vi "Actor Core.vi"(8 "error in":errorcluster, 11 "Autosampler in":refnum<class "Autosampler.lvclass">) -> (0 "error out":errorcluster, 3 "Actor out":refnum<class "Actor.lvclass">)   [LabVIEW 2023, in "Autosampler.lvlib" / "Autosampler.lvclass"]
doc: "(<B>Filename</B>: Actor Framework.lvlib:Actor.lvclass:Actor Core.vi)\n\nReceives messages to the actor, reacts to them, and initiates any error handling that may shut the actor down.\n\nDescendant classes may override this VI to append parallel tasks for the actor to complete while it handles messages. Overrides use the Call Parent Method node."
uses:
  Autosampler.lvclass
  Autosampler.lvclass/Autosampler.ctl
  Device/Device.lvclass
  <vilib>/ActorFramework/Actor/Actor.lvclass
  C:/FLASH/Development/Hardware/Device/Device.lvclass
  C:/Program Files/National Instruments/LabVIEW 2023/vi.lib/ActorFramework/Actor/Actor.lvclass
  C:/FLASH/Development/Hardware/Autosampler/Autosampler.lvclass
  Autosampler Messages/Status Update Msg/Status Update Msg.lvclass
  <vilib>/ActorFramework/Message Enqueuer/Message Priority.ctl
  <vilib>/ActorFramework/Message Enqueuer/Message Enqueuer.lvclass
panel:
  in  "Stop Button":bool
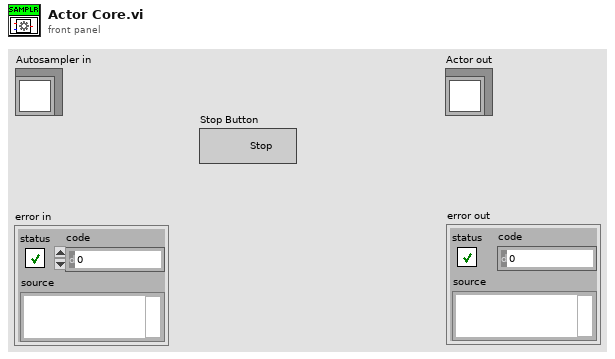
[diagram p1: front panel]
types:
  T1 = typedef "Actor Framework.lvlib/Message Enqueuer.lvclass/Message Priority.ctl" = enum16{"Low", "Normal", "High"}
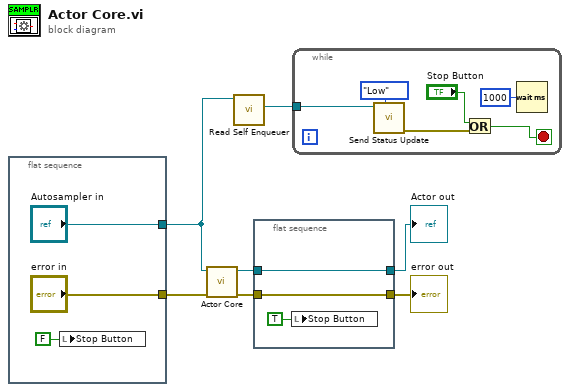
[diagram p0: block diagram]
diagram:
  n1 = flat-sequence {
    tunnel: ["error in"] -> w7
    tunnel: ["Autosampler in"] -> w2
    frame #0 {
      n2 = local write "Stop Button"(FALSE ("Stop Button")) -> ()
    }
  }
  n3 = call-parent "Actor Core.vi"("error in"=w7, "Device in"=w2) -> ("error out"=w3:errorcluster, "Actor out"=w6:refnum<class "Actor.lvclass">)  [unwired: 8 in]
  n4 = call <vilib>:"Read Self Enqueuer.vi"("Actor"=w2) -> ("Self Enqueuer"=w1:refnum<class "Message Enqueuer.lvclass">)  [unwired: 10 in]
  n5 = flat-sequence {
    tunnel: w6 -> [w12]
    tunnel: [w12] -> w5
    tunnel: [w11] -> w4
    tunnel: w3 -> [w11]
    frame #0 {
      n6 = local write "Stop Button"(TRUE ("Stop Button")) -> ()
    }
  }
  n7 = while {
    tunnel: w1 -> [w19]
    stop <- w15 stop-if-true
    n8 = call "Send Status Update.vi"("Message Priority (Normal)"=Message_Priority."Low", "Message Enqueuer"=w19) -> ("error out"=w16:errorcluster)  [unwired: 8 in, 1 out]
    n9 = Or(x="Stop Button", y=w16) -> (x .or. y?=w15:bool)
    n10 = Wait (ms)(milliseconds to wait=u32 1000 ("millisecond multiple")) -> ()  [unwired: 1 out]
  }
  "error out" <- w4
  "Actor out" <- w5
